vi "ESP_Scan_Code.vi"(0 "Offset":i32, 6 "steps between scans":sgl format="%.2f", 8 "total steps in line":i32=100, 9 "Axis":i32=1 min=1 max=4, 10 "lines per scan":i32=128, 11 "I/O chan for motor pulse":i32=7) -> (3 "Output String":string)   [LabVIEW 2022 SP3]
uses:
  -MotionRoutines/MotionGlobals.vi
panel:
  out "length":i32
  # "Not used anymore"
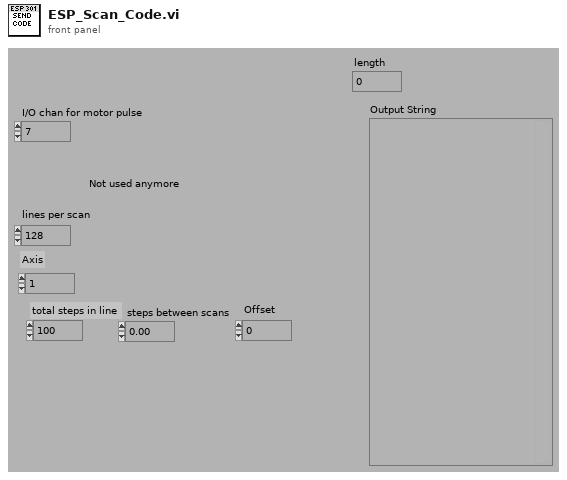
[diagram p1: front panel]
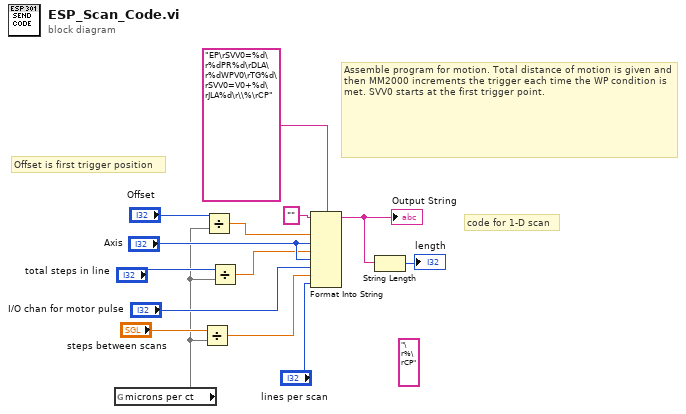
[diagram p0: block diagram]
diagram:
  (unwired) "\r%\rCP"
  # "Offset is first trigger position"
  # "code for 1-D scan"
  # "Assemble program for motion. Total distance of motion is given and\nthen MM2000 increments the trigger each time the WP condition is met. SVV0 starts at the first trigger point."
  n1 = global read "MotionGlobals.vi" "microns per ct"() -> (w3)
  n2 = Divide(x="steps between scans", y=w3) -> (x/y=w7:sgl)
  n3 = Divide(x="Offset", y=w3) -> (x/y=w2:dbl)
  n4 = Divide(x="total steps in line", y=w3) -> (x/y=w6:dbl)
  n5 = Format Into String(format string="EP\rSVV0=%d\r%dPR%d\rDLA\r%dWPV0\rTG%d\rSVV0=V0+%d\rJLA%d\r\\%\rCP", initial string="", w2, "Axis", w6, "Axis", "I/O chan for motor pulse", w7, "lines per scan") -> (resulting string=w1:string)  [unwired: 1 in, 1 out]
  "Output String" <- w1
  n6 = String Length(string=w1) -> (length=→"length":i32)
